vi "VRMSFreqConfigurationSubVI.vi"(8 "error in":errorcluster, 10 "Sim?":bool, 11 "physical channel":tag) -> (0 "error out":errorcluster, 3 "task out":refnum<k21>)   [LabVIEW 2017]
uses:
  <vilib>/DAQmx/configure/timing.llb/DAQmx Timing (Sample Clock).vi
  <vilib>/DAQmx/create/channels.llb/DAQmx Create Channel (AI-Voltage-Basic).vi
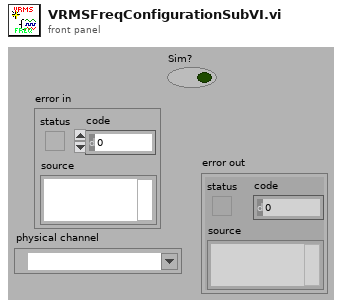
[diagram p1: front panel]
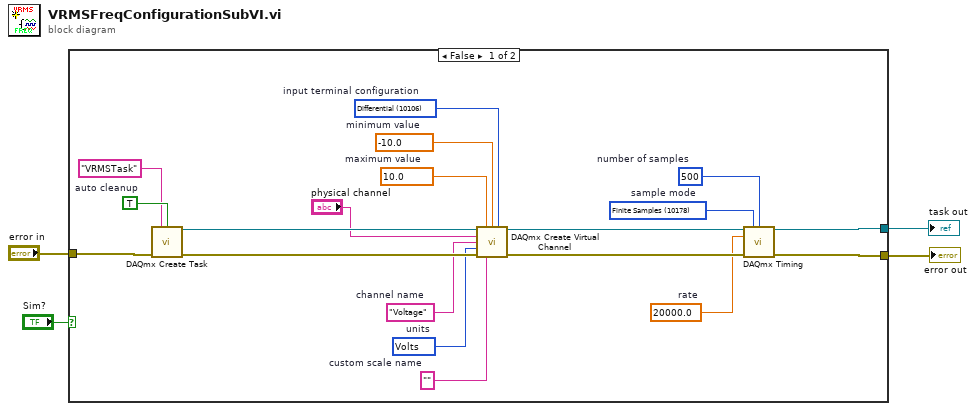
[diagram p0: block diagram]
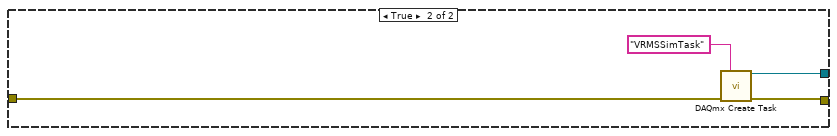
[diagram p2: hidden frame]
diagram:
  n1 = case shown="False" "Sim?" {
    tunnel: "error in" -> [w23 w27]
    tunnel: [w12 w25] -> w3
    tunnel: [w11 w26] -> w2
    frame False {
      w7 = 10178 items=["Finite Samples"=10178, "Continuous Samples"=10123, "Hardware Timed Single Point"=12522]  # sample mode
      w8 = 500  # number of samples
      w9 = 20000.0  # rate
      w13 = 10106 items=["default"=-1, "RSE"=10083, "NRSE"=10078, "Differential"=10106, "Pseudodifferential"=12529]  # input terminal configuration
      w14 = 10348 items=["Volts"=10348, "From Custom Scale"=10065]  # units
      w15 = "Voltage"  # channel name
      w17 = ""  # custom scale name
      w18 = -10.0  # minimum value
      w19 = 10.0  # maximum value
      w21 = TRUE  # auto cleanup
      n2 = call <vilib>:"DAQmx Create Task.vi"("new task name"="VRMSTask", "auto cleanup"=w21, "error in"=w23) -> ("task out"=w20:refnum<k21>, "error out"=w22:errorcluster)  [unwired: 11 in]
      n3 = call-poly <vilib>:"DAQmx Create Virtual Channel.vi"("task in"=w20, "maximum value"=w19, "minimum value"=w18, "input terminal configuration"=w13, "physical channels"="physical channel", "name to assign"=w15, "units"=w14, "error in"=w22, "custom scale name"=w17) -> ("task out"=w10:refnum<k21>, "error out"=w16:errorcluster)  [unwired: 5 in]
      n4 = call-poly <vilib>:"DAQmx Timing.vi"("task/channels in"=w10, "sample mode"=w7, "samples per channel"=w8, "rate"=w9, "error in"=w16) -> ("task out"=w12:refnum<k21>, "error out"=w11:errorcluster)  [unwired: 9 in]
    }
    frame True {
      n5 = call <vilib>:"DAQmx Create Task.vi"("new task name"="VRMSSimTask", "error in"=w27) -> ("task out"=w25:refnum<k21>, "error out"=w26:errorcluster)  [unwired: 12 in]
    }
  }
  "error out" <- w2
  "task out" <- w3
